vi "MessageForLooser.vi"(11 "String in":string) -> (3 "String out":string)   [LabVIEW 2020]
doc: "Parse description for fail ending."
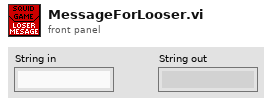
[diagram p1: front panel]
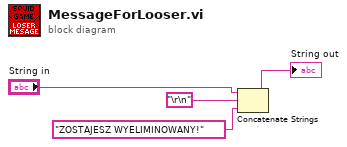
[diagram p0: block diagram]
diagram:
  n1 = Concatenate Strings("String in", "\r\n", "ZOSTAJESZ WYELIMINOWANY!" ("T button name (\"OK\")")) -> (→"String out":string)
